vi "ELM(TCP) - labview 2015.vi"() -> ()   [LabVIEW 2015]
doc: "The Basic Serial Read and Write example performs a Serial Port Read, a Serial Port Write, or a combination of these actions. The user selects the actions (read or write) on the front panel. If both are selected, the VI will write the data first, read data, and then close the VISA session that is opened to the port. This VI will wait until the specified number of bytes is received at the port or until a termination character is read.\n\nINSTRUCTIONS:\n1) Select the serial resource and configuration parameters (baud rate, data bits, parity, stop bits, flow control).\n2) Select the operations to be performed. \n3) Connect the serial port to your device. If no device is available, perform a loopback test by doing one of the following. Short pins 2 and 3 on a RS-232 cable or short pin 4 to pin 8 and pin 5 to pin 9 on a RS-485/422 cable. \n4) Run the VI to see the data read. (The \"read string\" will match the \"string to write\" if a loopback test was performed.)\n\nNote: The parameters set for the serial port must match the parameters of the connected instrument or device. In this example, the bytes to read parameter specifies the number of bytes that the serial port reads. If there were more bytes at the port than the number specified in bytes to read, those bytes would not be read. Also, if you specify to read more bytes than the number of bytes actually read, you might receive a timeout error message.\n\nOn the block diagram, the Configure Serial Port VI sets the configuration parameters. The front panel displays the controls used to configure the basic parameters, such as baud rate, data bits, and parity. Constants configure the other parameters the user probably does not need set. After the VISA Configure Serial Port VI opens the VISA session and configures the port, the VI passes the VISA resource name to other VIs that perform operations on that VISA resource. The VISA Write function sends a command to the serial device and the VISA Read function returns data based on the command. The VISA Close function then closes the reference to the serial device. It is important to close the reference; otherwise communication through with that port through protocols other than VISA might not be possible."
uses:
  <vilib>/Platform/TimedLoop/XDataNode/timing_clust.ctl
  <vilib>/Platform/TimedLoop/XDataNode/nitl_modes.ctl
  <vilib>/Platform/TimedLoop/XDataNode/wakeup.ctl
  <vilib>/Utility/file.llb/Write Delimited Spreadsheet (DBL).vi
  <vilib>/platform/TimedLoop/XDataNode/XDataNode.xnode
  <vilib>/Platform/TimedLoop/XDataNode/XDNodeRunTimeDep.lvlib
panel:
  out "?":dbl[](array[numeric])
  out "?":dbl[](array[numeric])
  out "?":dbl[](array[numeric])
  out "?":dbl[](array[numeric])
  out "?":dbl[](array[numeric])
  out "?":dbl[](array[numeric])
  out "?":dbl[](array[numeric])
  out "?":dbl[](array[numeric])
  in  "CAMINHO DO ARQUIVO DE AQUISIÇÃO DE DADOS":path
  out "TEMPO DE EXECUÇÃO DA LEITURA":dbl[](array[numeric])
  out "Tempo(s)":dbl
  out "?":dbl[](array[numeric])
  out "RESPOSTA ELM327":string
  in  "?":bool=TRUE
  in  "?":string="*IDN?\n"
  in  "?":bool
  in  "?":i32
  in  "?":u16
  in  "?":string
  in  "?":u32=500
  out "CONTADOR 9":dbl
  out "Vazão do ar":dbl(graph)
  out "CONTADOR 8":dbl
  out "Posição da\nborboleta":dbl(graph)
  out "CONTADOR 7":dbl
  out "Nível de\ncombustível":dbl(graph)
  out "CONTADOR 6":dbl
  out "Tensão da\nbateria":dbl(graph)
  out "CONTADOR 5":dbl
  out "Pressão absoluta\ndo coletor":dbl(graph)
  out "CONTADOR 4":dbl
  out "Temperatura\ndo ar de admissão":dbl(graph)
  out "CONTADOR 3":dbl
  out "Velocidade":dbl(graph)
  out "CONTADOR 1":dbl
  out "Temperatura\ndo fluido de\narrefecimento":dbl(graph)
  out "CONTADOR 2":dbl
  out "RPM":dbl(graph)
  in  "?":bool
  # "Processo de conexão e aplicação do código"
  # "Painel de Aquisição dos Dados"
  # "ATZ\nATI\nATE0\nATL0\nATS0\nATH0\nATSP0\nATDP\nATRV\nATDPN"
  # "Reinicia o ELM327\nIdentificação do ELM327\nDesabilita eco\nRemove Line Feed\nRemove espaços\nOculta cabeçalhos\nSeleção automática do protocolo\nMostra o protocolo utilizado\nLê a tensão da bateria\nNúmero do protocolo atual"
  # "PID'S DE DIAGNÓSTICO\n        AUTOMOTIVO"
  # "Após conectar o OBD II ao computador, informe o endereço IP do adaptador ELM327 Wi-Fi. Os endereços mais comuns são 192.168.0.10 e 192.168.0.11. Utilize um tempo de espera antes da leitura entre 500 ms e 1000 ms. Para a porta TCP, utilize preferencialmente a porta 35000. Para o número de bytes de leitura, recomenda-se utilizar 100 bytes. Execute os comandos AT antes da leitura dos PIDs para configurar o ELM327 e obter respostas mais limpas e consistentes. Após essa configuração, realize a leitura dos PIDs desejados."
  # "0105\n010C\n010D\n010F\n0110\n0111\n010B\n0142\n012F\n0100"
  # "Temperatura do fluido de arrefecimento\nRPM do motor\nVelocidade do veículo\nTemperatura do ar de admissão\nVazão de ar\nPosição da borboleta\nPressão absoluta do coletor\nTensão do módulo de controle\nNível de combustível\nPIDs suportados"
  # "Gráficos dos PID's no domínio do  tempo"
  # "Link do GITHUB para acessar este trabalho:"
  # "https://github.com/tiagod-mxavier/meus-trabalhos/tree/main"
  # "Nível de combustível"
  # "Temperatura do ar\nde admissão"
  # "Tensão do módulo de controle"
  # "Pressão absoluta do coletor"
  # "Posição da borboleta"
  # "Vazão de ar"
  # "Velocidade do veículo"
  # "RPM do motor"
  # "Temperatura do fluido\nde arrefecimento"
  # "ANÁLISE DO DESEMPENHO DO MOTOR FORD ZETEC 1.8"
  # "ENTRADA"
  # "EXECUÇÃO"
  # "ENDEREÇO IP"
  # "TEMPO DE ESPERA ANTES DA LEITURA"
  # "PORTA TCP"
  # "Nº DE BYTES\nP/ LEITURA"
  # "COMANDOS ÚTEIS PARA\n     INÍCIO DE LEITURA"
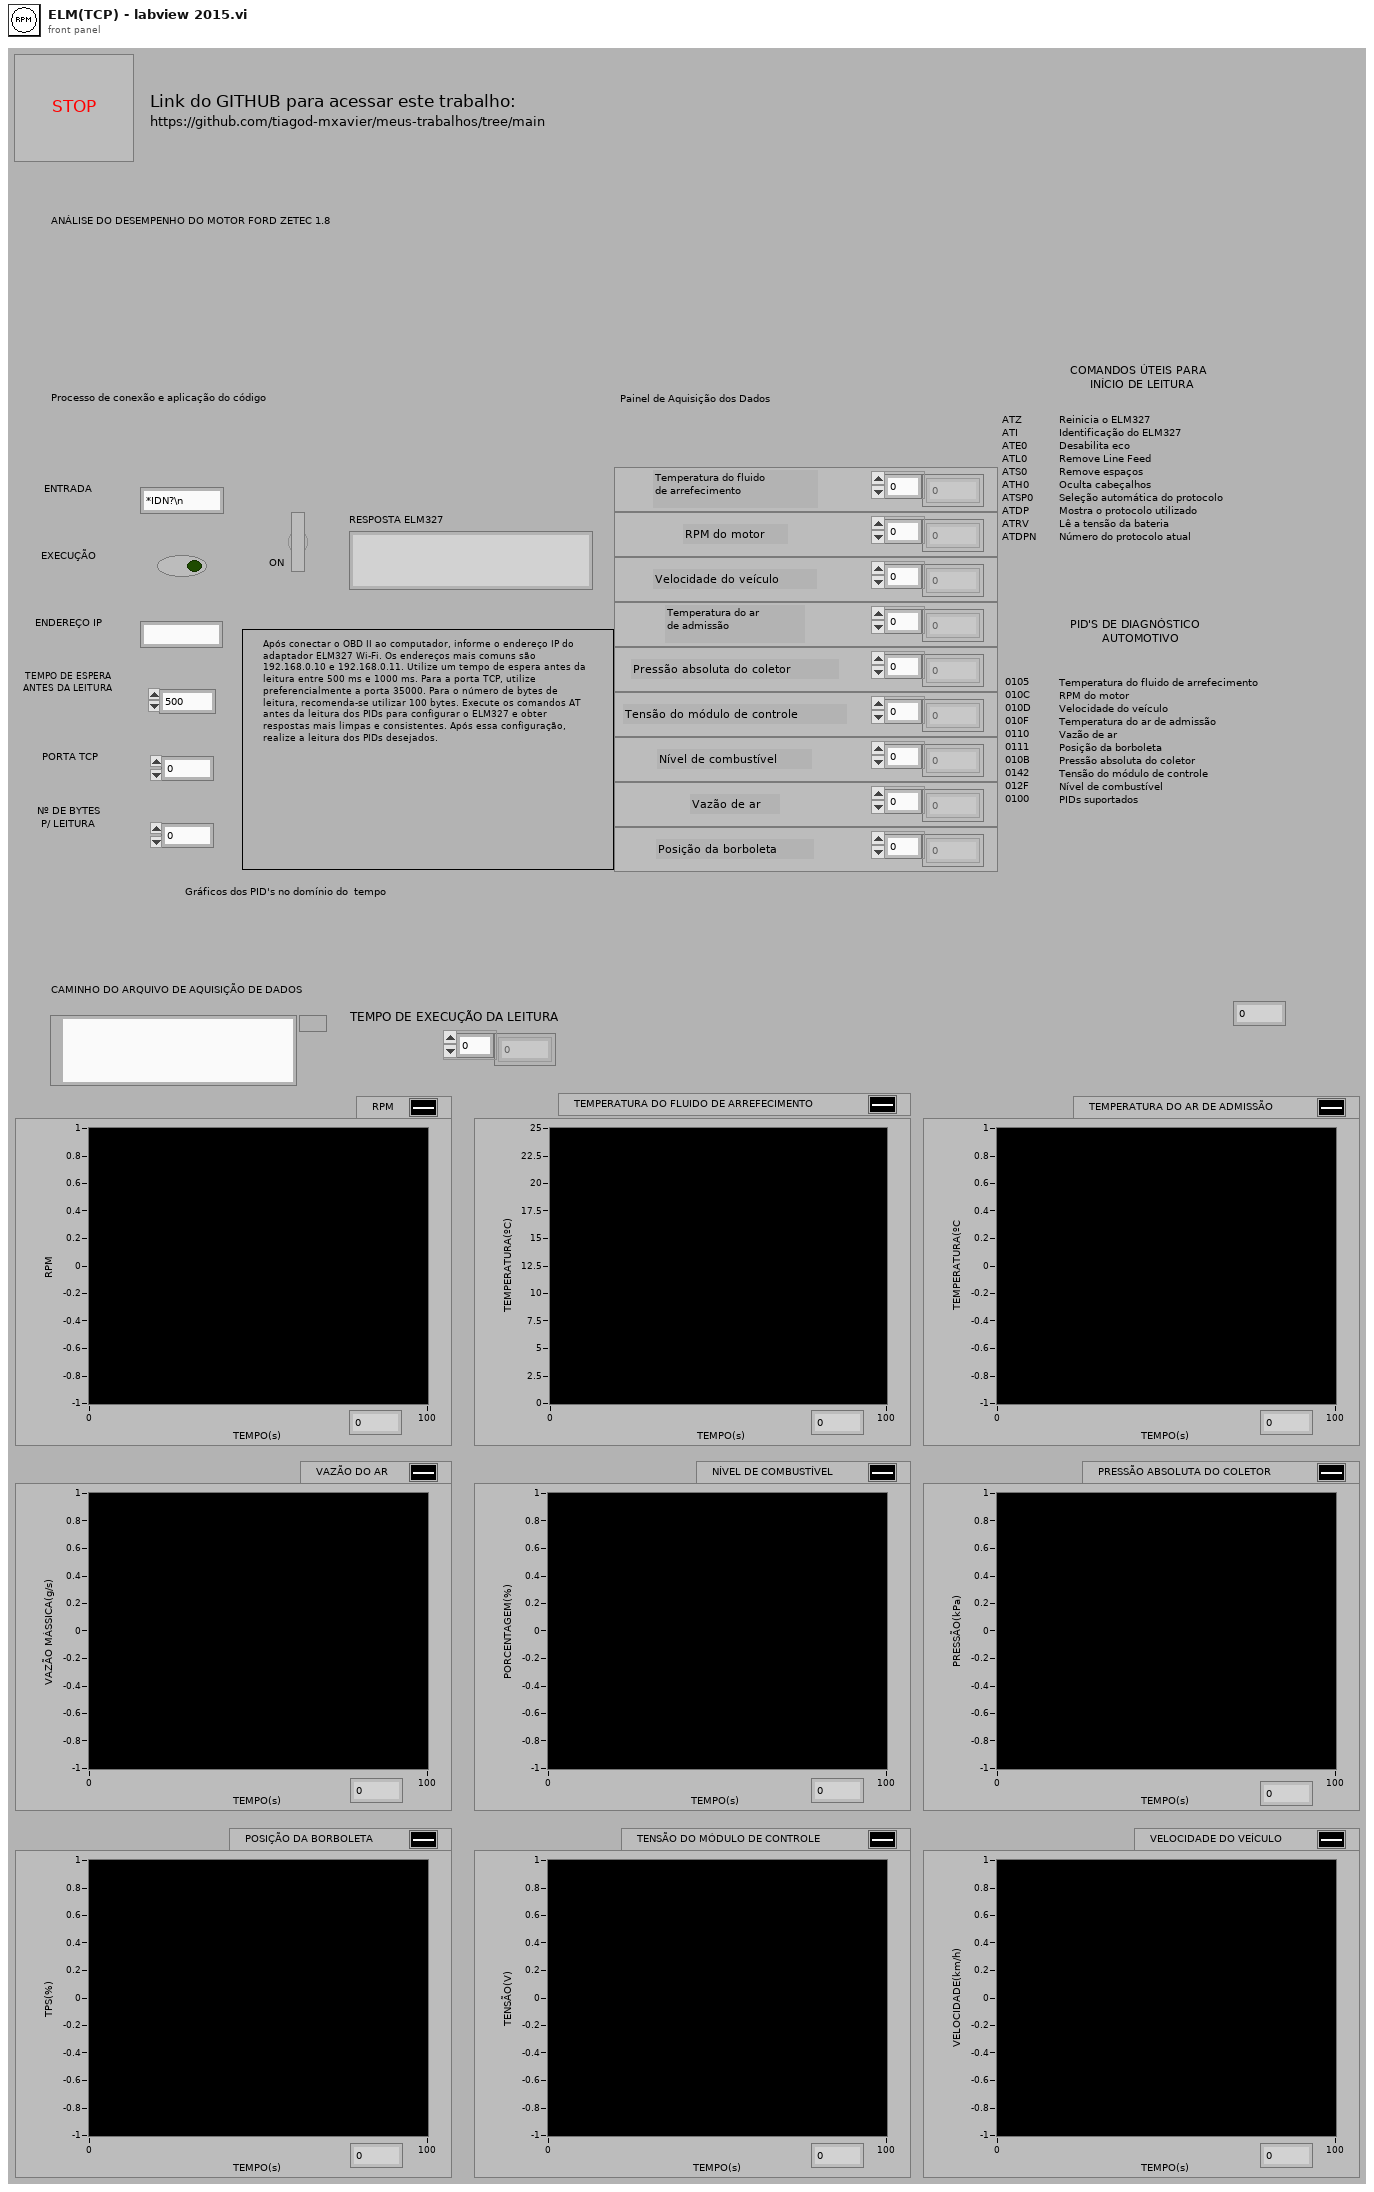
[diagram p1: front panel]
types:
  T1 = typedef "XDNodeRunTimeDep.lvlib/timing_clust.ctl" = cluster{"Expected End [f-1]":u64, "Actual End [f-1]":u64, "Finished Late? [f-1]":bool, "Expected End [i-1]":u64, "Actual End [i-1]":u64, "Finished Late? [i-1]":bool, "Expected Start [i]":u64, "Actual Start [i]":u64, "Expected Start [f]":u64, "Actual Start [f]":u64, "Source Name":string, "Structure Name":string, "Period":i64, "Deadline":i64, "Offset":i64, "Start":i64, "Priority":i32, "Timeout":i32, "Mode":T2, "Wakeup Reason":T3, "Error":errorcluster, "Source Type":string, "Secondary Source Type":string, "Global End Time":u64, "Global Start Time":u64, "Frame Duration":u64, "Iteration Duration":u64, "Assigned CPU":i32, "I/O Scan Engine Mode":u32}
  T2 = typedef "XDNodeRunTimeDep.lvlib/nitl_modes.ctl" = enum32{"No Change", "Process missed periods, maintain original phase", "Discard missed periods, maintain original phase", "Process missed periods, ignore original phase", "Discard missed periods, ignore original phase"}
  T3 = typedef "XDNodeRunTimeDep.lvlib/wakeup.ctl" = enum32{"Normal", "Aborted", "Asynchronous wakeup", "Timing source error", "Timed loop error", "Timeout"}
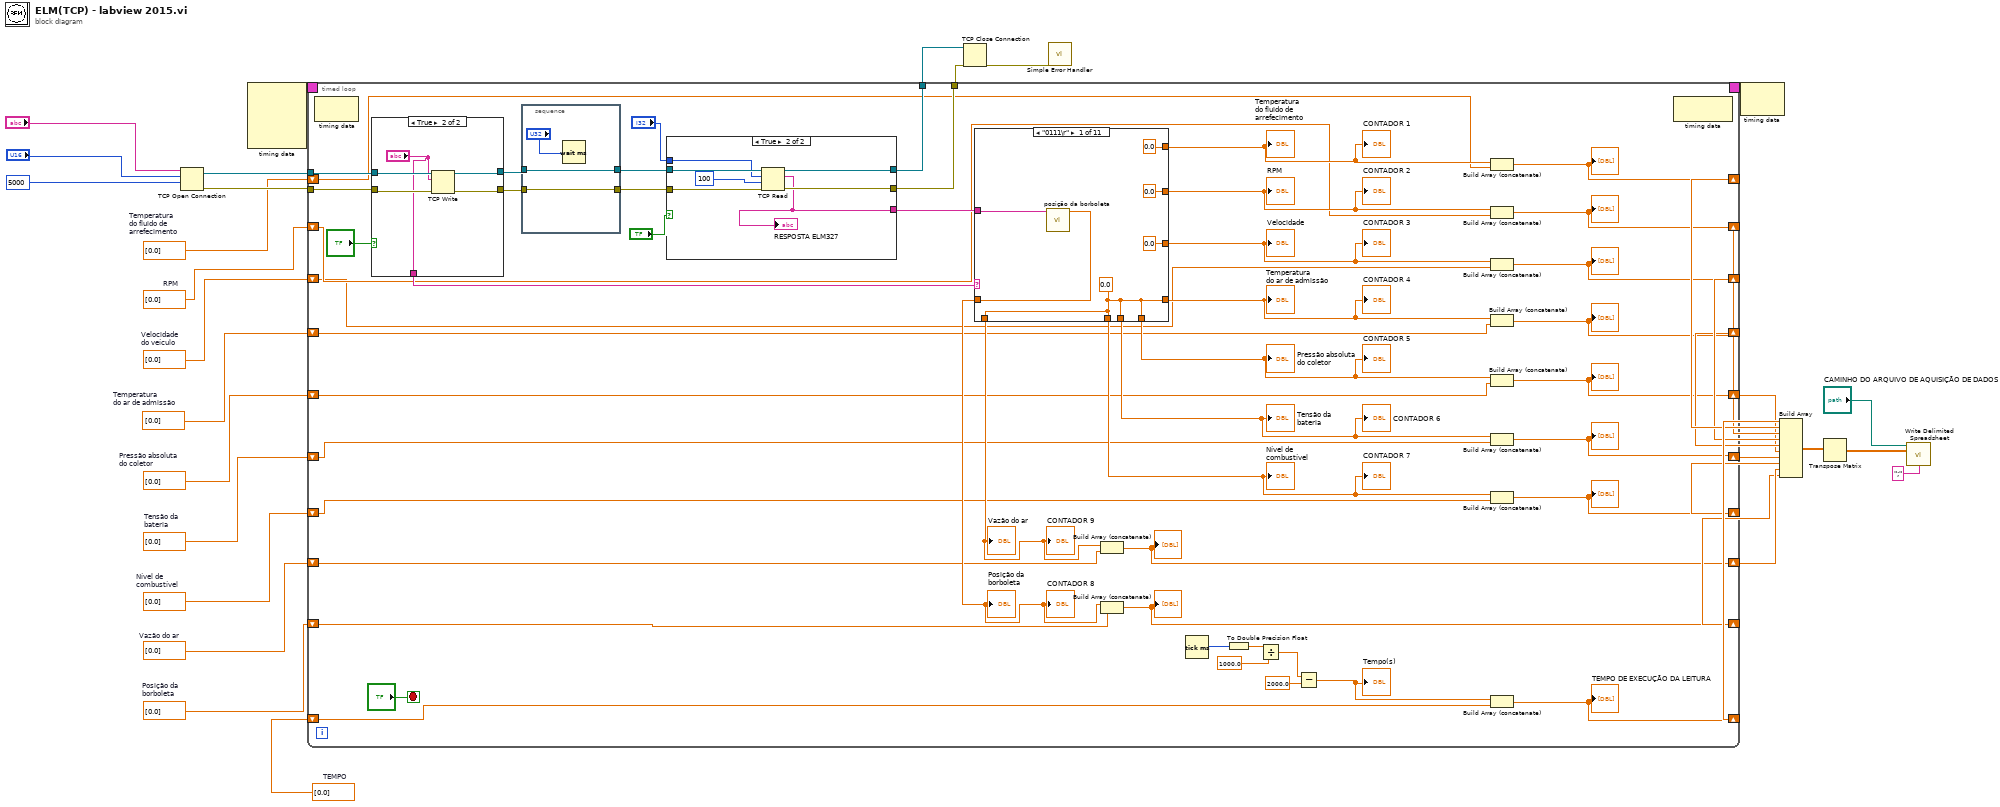
[diagram p0: block diagram]
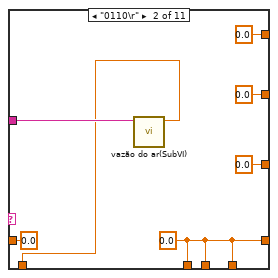
[diagram p2: hidden frame]
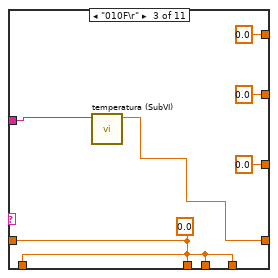
[diagram p3: hidden frame]
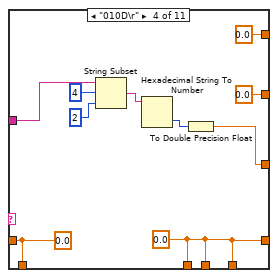
[diagram p4: hidden frame]
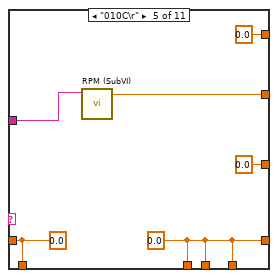
[diagram p5: hidden frame]
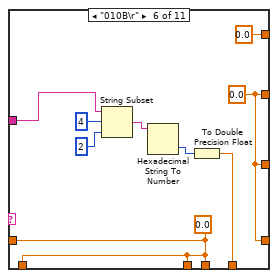
[diagram p6: hidden frame]
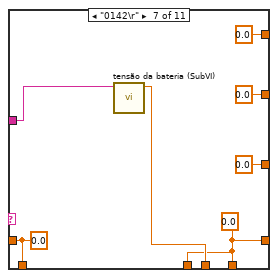
[diagram p7: hidden frame]
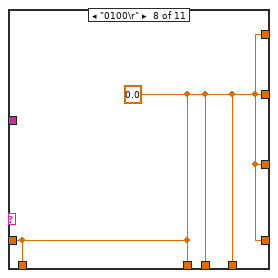
[diagram p8: hidden frame]
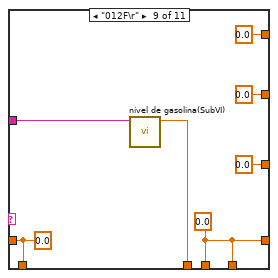
[diagram p9: hidden frame]
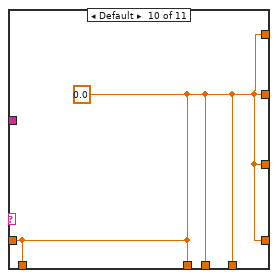
[diagram p10: hidden frame]
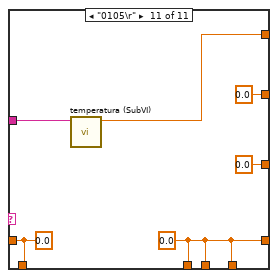
[diagram p11: hidden frame]
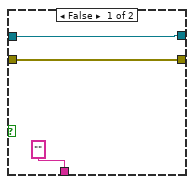
[diagram p12: hidden frame]
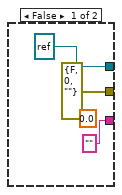
[diagram p13: hidden frame]
diagram:
  w16 = dbl[] [0.0]  # Posição da borboleta
  w17 = dbl[] [0.0]  # Vazão do ar
  w15 = dbl[] [0.0]  # Nível de combustível
  w18 = dbl[] [0.0]  # Tensão da bateria
  w19 = dbl[] [0.0]  # Pressão absoluta do coletor
  w20 = dbl[] [0.0]  # Temperatura do ar de admissão
  w21 = dbl[] [0.0]  # RPM
  w22 = dbl[] [0.0]  # Velocidade do veículo
  w23 = dbl[] [0.0]  # TEMPO
  w24 = dbl[] [0.0]  # Temperatura do fluido de arrefecimento
  n1 = TCP Open Connection(address="?", remote port or service name="?", timeout ms (60000)=5000) -> (connection ID=w29:refnum<k5>, error out=w28:errorcluster)  [unwired: 2 in]
  n2 = node-c288() -> (w34:T1)  [unwired: 4 in]
  n3 = timed-loop {
    timing: w34 -> [_]
    timing-out: [_] -> w33
    tunnel: w29 -> [w80]
    tunnel: w28 -> [w81]
    tunnel: [w73] -> w27
    tunnel: [w72] -> w26
    shift-right: [w68] -> w13
    shift-left: w24 -> [w47]
    shift-right: [w52] -> w14
    shift-left: w23 -> [w46]
    shift-right: [w63] -> w11
    shift-left: w22 -> [w41]
    shift-right: [w61] -> w12
    shift-left: w21 -> [w42]
    shift-right: [w59] -> w10
    shift-left: w20 -> [w40]
    shift-right: [w58] -> w9
    shift-left: w19 -> [w39]
    shift-right: [w55] -> w8
    shift-left: w18 -> [w38]
    shift-right: [w53] -> w7
    shift-left: w15 -> [w37]
    shift-right: [w49] -> w6
    shift-left: w17 -> [w36]
    shift-right: [w48] -> w5
    shift-left: w16 -> [w35]
    stop <- "?" stop-if-true
    n4 = node-c288() -> ()  [unwired: 1 in, 1 out]
    n5 = case shown="True" "?" {
      tunnel: [w152 w157] -> w83
      tunnel: [w151 w156] -> w82
      tunnel: w81 -> [w151 w155]
      tunnel: w80 -> [w152 w154]
      tunnel: ["" "?"] -> w70
      frame False {
      }
      frame True {
        n6 = TCP Write(connection ID=w154, data in="?", error in (no error)=w155) -> (connection ID out=w157:refnum<k5>, error out=w156:errorcluster)  [unwired: 1 in, 1 out]
      }
    }
    n7 = stacked-sequence {
      tunnel: w83 -> [w169]
      tunnel: w82 -> [w168]
      tunnel: [w169] -> w79
      tunnel: [w168] -> w78
      frame #0 {
        n8 = Wait (ms)(milliseconds to wait="?") -> ()  [unwired: 1 out]
      }
    }
    n9 = case shown="True" "?" {
      tunnel: w79 -> [_ w165]
      tunnel: w78 -> [_ w164]
      tunnel: [errorcluster {"status"=FALSE, "code"=0, "source"=""} ("error out") w167] -> w72
      tunnel: [refnum<k5> refnum ("connection ID") w166] -> w73
      tunnel: "?" -> [_ w162]
      tunnel: ["" ("data out") w161] -> w71
      frame False {
        (unwired) 0.0 ("Numeric")
        (unwired) 0.0
        (unwired) 0.0
      }
      frame True {
        n10 = TCP Read(connection ID=w165, bytes to read=w162, error in (no error)=w164, 9:100 ("timeout ms (25000)")) -> (connection ID out=w166:refnum<k5>, data out=w161:string, error out=w167:errorcluster)  [unwired: 1 in]
        "RESPOSTA ELM327" <- w161
      }
    }
    n11 = case shown="\"0111\\r\"" w70 {
      tunnel: w71 -> [w84 w96 w102 w112 w118 w123 w134 _ w142 _ w149]
      tunnel: [0.0 ("Numeric") 0.0 ("Numeric") 0.0 ("Numeric") 0.0 ("Numeric") 0.0 ("Numeric") 0.0 ("Numeric") 0.0 ("Numeric") w135 0.0 ("Numeric") w143 w148] -> w69
      tunnel: [0.0 ("Numeric") 0.0 ("Numeric") 0.0 ("Numeric") 0.0 ("Numeric") w117 w120 0.0 ("Numeric") w135 0.0 ("Numeric") w143 0.0 ("Numeric")] -> w62
      tunnel: [0.0 ("Numeric") 0.0 0.0 w107 0.0 w120 0.0 ("Numeric") w135 0.0 ("Numeric") w143 0.0 ("Numeric")] -> w64
      tunnel: [w89 w91 w101 w106 w114 w120 w129 w135 w137 w143 w146] -> w60
      tunnel: [w89 w91 w97 w106 w114 w122 w129 w135 w137 w143 w146] -> w56
      tunnel: [w89 w91 w97 w106 w114 w119 w133 w135 w137 w143 w146] -> w57
      tunnel: [w89 w91 w97 w106 w114 w119 w129 w135 w141 w143 w146] -> w54
      tunnel: [w89 w95 w97 w105 w113 w119 w128 w135 w136 w143 w147] -> w51
      tunnel: [w85 0.0 ("Numeric") w97 w105 w113 w119 w128 w135 w136 w143 w147] -> w50
      frame "0111\r" {
        w89 = 0.0 ("Numeric")
        n12 = call "posição da borboleta.vi"("data in"=w84) -> ("Numeric"=w85:dbl)  [unwired: 10 in]
      }
      frame "0110\r" {
        w91 = 0.0 ("Numeric")
        n13 = call "vazão do ar(SubVI).vi"("data in"=w96) -> ("Numeric"=w95:dbl)  [unwired: 10 in]
      }
      frame "010F\r" {
        w97 = 0.0 ("Numeric")
        n14 = call "temperatura (SubVI).vi"("data in"=w102) -> ("Numeric"=w101:dbl)  [unwired: 10 in]
      }
      frame "010D\r" {
        w105 = 0.0 ("Numeric")
        w106 = 0.0 ("Numeric")
        n15 = String Subset(string=w112, offset (0)=4, length (rest)=2 ("length (rest)")) -> (substring=w109:string)
        n16 = Hexadecimal String To Number(string=w109) -> (number=w108:u32)  [unwired: 2 in, 1 out]
        n17 = To Double Precision Float(number=w108) -> (double precision float=w107:dbl)
      }
      frame "010C\r" {
        w113 = 0.0 ("Numeric")
        w114 = 0.0 ("Numeric")
        n18 = call "RPM (SubVI).vi"("data in"=w118) -> ("Numeric"=w117:dbl)  [unwired: 10 in]
      }
      frame "010B\r" {
        w119 = 0.0 ("Numeric")
        w120 = 0.0 ("Numeric")
        n19 = String Subset(string=w123, offset (0)=4, length (rest)=2 ("length (rest)")) -> (substring=w125:string)
        n20 = Hexadecimal String To Number(string=w125) -> (number=w124:u32)  [unwired: 2 in, 1 out]
        n21 = To Double Precision Float(number=w124) -> (double precision float=w122:dbl)
      }
      frame "0142\r" {
        w128 = 0.0 ("Numeric")
        w129 = 0.0 ("Numeric")
        n22 = call "tensão da bateria (SubVI).vi"("data in"=w134) -> ("Numeric"=w133:dbl)  [unwired: 10 in]
      }
      frame "0100\r" {
        w135 = 0.0 ("Numeric")
      }
      frame "012F\r" {
        w137 = 0.0 ("Numeric")
        w136 = 0.0 ("Numeric")
        n23 = call "nível de gasolina(SubVI).vi"("data in"=w142) -> ("Numeric"=w141:dbl)  [unwired: 10 in]
      }
      frame Default {
        w143 = 0.0 ("Numeric")
      }
      frame "0105\r" {
        w146 = 0.0 ("Numeric")
        w147 = 0.0 ("Numeric")
        n24 = call "temperatura (SubVI).vi"("data in"=w149) -> ("Numeric"=w148:dbl)  [unwired: 10 in]
      }
    }
    "RPM" <- w62
    "CONTADOR 2" <- w62
    "Temperatura\ndo fluido de\narrefecimento" <- w69
    "CONTADOR 1" <- w69
    "Velocidade" <- w64
    "CONTADOR 3" <- w64
    "Temperatura\ndo ar de admissão" <- w60
    "CONTADOR 4" <- w60
    "Pressão absoluta\ndo coletor" <- w56
    "CONTADOR 5" <- w56
    "Tensão da\nbateria" <- w57
    "CONTADOR 6" <- w57
    "Nível de\ncombustível" <- w54
    "CONTADOR 7" <- w54
    "Posição da\nborboleta" <- w50
    "CONTADOR 8" <- w50
    "Vazão do ar" <- w51
    "CONTADOR 9" <- w51
    n25 = Build Array (concatenate)(w51, w36) -> (w49:dbl[])
    "?" <- w49
    n26 = Build Array (concatenate)(w50, w35) -> (w48:dbl[])
    "?" <- w48
    n27 = Tick Count (ms)() -> (millisecond timer value=w67:u32)
    n28 = To Double Precision Float(number=w67) -> (double precision float=w66:dbl)
    n29 = Divide(x=w66, y=1000.0) -> (x/y=w45:dbl)
    n30 = Subtract(x=w45, y=2000.0) -> (x-y=w44:dbl)
    "Tempo(s)" <- w44
    n31 = Build Array (concatenate)(w69, w47) -> (w68:dbl[])
    "?" <- w68
    n32 = Build Array (concatenate)(w62, w42) -> (w61:dbl[])
    "?" <- w61
    n33 = Build Array (concatenate)(w64, w41) -> (w63:dbl[])
    "?" <- w63
    n34 = Build Array (concatenate)(w60, w40) -> (w59:dbl[])
    "?" <- w59
    n35 = Build Array (concatenate)(w56, w39) -> (w58:dbl[])
    "?" <- w58
    n36 = Build Array (concatenate)(w57, w38) -> (w55:dbl[])
    "?" <- w55
    n37 = Build Array (concatenate)(w54, w37) -> (w53:dbl[])
    "?" <- w53
    n38 = Build Array (concatenate)(w44, w46) -> (w52:dbl[])
    "TEMPO DE EXECUÇÃO DA LEITURA" <- w52
    n39 = node-c288() -> ()  [unwired: 1 in, 1 out]
  }
  n40 = TCP Close Connection(connection ID=w27, error in (no error)=w26) -> (error out=w25:errorcluster)  [unwired: 1 in, 1 out]
  n41 = call <vilib>:"Simple Error Handler.vi"("error in (no error)"=w25) -> ()  [unwired: 1 in, 8 out]
  n42 = node-c288(w33) -> ()  [unwired: 1 out]
  n43 = Build Array(w14, w13, w12, w11, w10, w9, w8, w7, w6, w5) -> (w4:dbl[][])
  n44 = Transpose Matrix(1:w4) -> (0:w3:dbl[][])
  n45 = call-poly <vilib>:"Write Delimited Spreadsheet.vi"("file path (dialog if empty)"="CAMINHO DO ARQUIVO DE AQUISIÇÃO DE DADOS", "2D data"=w3, "delimiter (\\t)"=";" ("delimiter (\\t)")) -> ()  [unwired: 11 in, 2 out]
